vi "tb_push and pop random sequence.vi"(9 "fifo depth":u8(ring)=10 items=["4"=2, "8"=3, "16"=4, "32"=5, "64"=6, "128"=7, "256"=8, "512"=9, "1024"=10, "2048"=11, "4096"=12, "8192"=13, "16384"=14, "32768"=15, "65536"=16, "131072"=17, "262144"=18, "524288"=19, "1048576"=20, "2097152"=21, "4194304"=22, "8388608"=23, "16777216"=24, "33554432"=25, "67108864"=26, "134217728"=27, "268435456"=28, "536870912"=29, "1073741824"=30, "2147483648"=31, "4294967296"=32], 10 "arbiter configuration":T1={"write grant time (clocks)"=100, "read grant time (clocks)"=100}, 11 "Memory":T2={"fifo1 memory"="Bank0", "fifo2 memory"="Bank1"}) -> (3 "Pass?":bool=TRUE)   [LabVIEW 2011]
uses:
  Data Type (256).ctl
  <instrlib>/RF-RIO/Memory/FPGA/Interface/Timeslot Arbiter Configuration.ctl
  <instrlib>/RF-RIO/Memory/FPGA/Memory.lvlib
panel:
  out "Iteration":i32
  out "FIFO Input":T3[](array[typedef])
  out "FIFO Output":T3[](array[typedef])
  # "Debug Area"
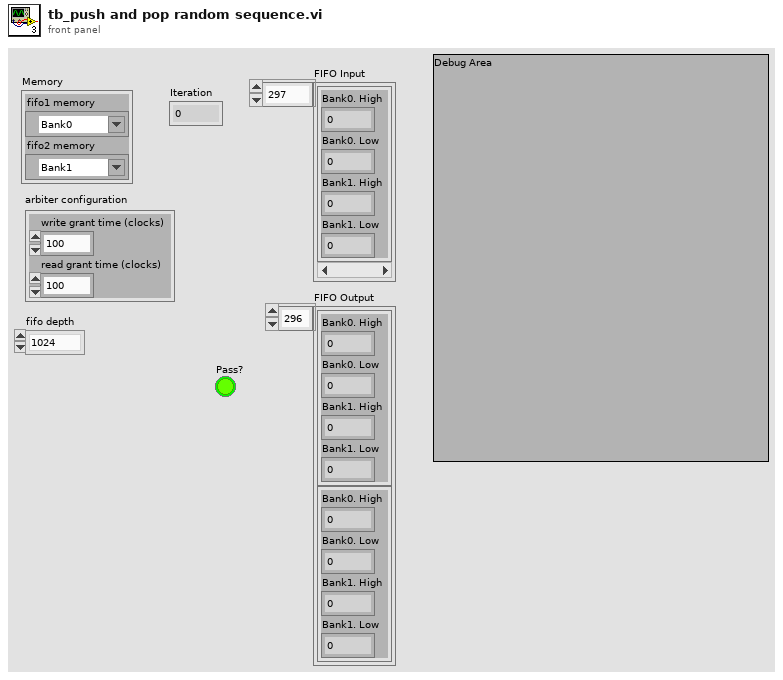
[diagram p1: front panel]
types:
  T1 = typedef "Memory.lvlib/Timeslot Arbiter Configuration.ctl" = cluster{"write grant time (clocks)":u16, "read grant time (clocks)":u16}
  T2 = cluster{"fifo1 memory":refnum<k21>, "fifo2 memory":refnum<k21>}
  T3 = typedef "Data Type (256).ctl" = cluster{"Bank0. High":u64, "Bank0. Low":u64, "Bank1. High":u64, "Bank1. Low":u64}
  T4 = cluster{"Bank0. High":bool, "Bank0. Low":bool, "Bank1. High":bool, "Bank1. Low":bool}[]
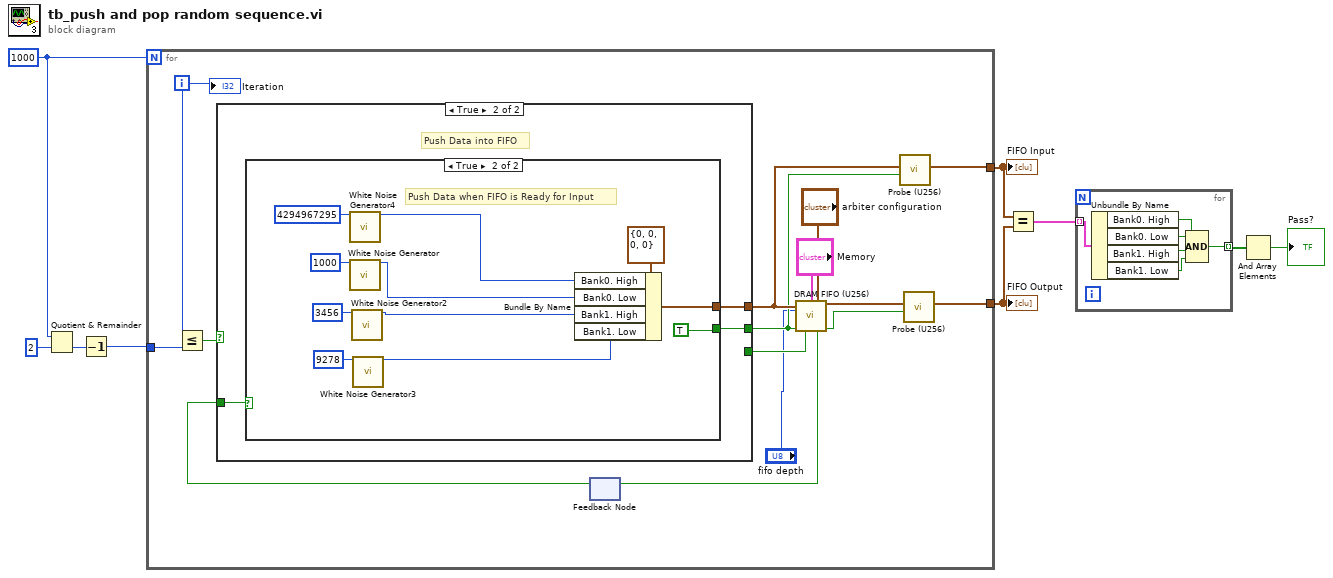
[diagram p0: block diagram]
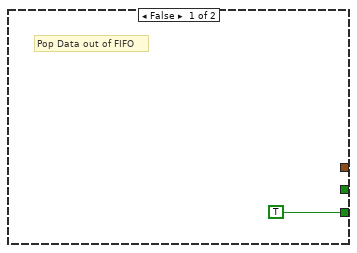
[diagram p2: hidden frame]
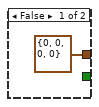
[diagram p3: hidden frame]
diagram:
  w9 = 1000
  n1 = Quotient & Remainder(x=w9, y=2) -> (floor(x/y)=w7:i32)  [unwired: 1 out]
  n2 = Decrement(x=w7) -> (x-1=w6:i32)
  n3 = for {
    N: w9 -> [_]
    tunnel: [w20] -> w4
    tunnel: [w17] -> w5
    tunnel: w6 -> [w14]
    i -> [w15]
    n4 = Less Or Equal?(x=w15, y=w14) -> (x <= y?=w16:bool)
    n5 = feedback #1() -> (w22:bool)  [unwired: 1 in]
    n6 = case shown="True" w16 {
      tunnel: [_ w28] -> w19
      tunnel: [_ w27] -> w18
      tunnel: w22 -> [_ w26]
      tunnel: [TRUE _] -> w21
      frame False {
        # "Pop Data out of FIFO"
      }
      frame True {
        # "Push Data into FIFO"
        n7 = case shown="True" w26 {
          tunnel: [T3 {"Bank0. High"=0, "Bank0. Low"=0, "Bank1. High"=0, "Bank1. Low"=0} ("Input Data") w39] -> w28
          tunnel: [_ TRUE] -> w27
          frame False {
          }
          frame True {
            # "Push Data when FIFO is Ready for Input"
            n8 = call "White Noise Generator4"("seed"=u32 4294967295) -> ("white noise out"=w30:i16)  [unwired: 14 in]
            n9 = call "White Noise Generator"("seed"=u32 1000) -> ("white noise out"=w31:i16)  [unwired: 14 in]
            n10 = call "White Noise Generator2"("seed"=u32 3456) -> ("white noise out"=w32:i16)  [unwired: 14 in]
            n11 = call "White Noise Generator3"("seed"=u32 9278) -> ("white noise out"=w33:i16)  [unwired: 14 in]
            n12 = Bundle By Name(cluster=T3 {"Bank0. High"=0, "Bank0. Low"=0, "Bank1. High"=0, "Bank1. Low"=0} ("Input Data"), "Bank0. High"=w30, "Bank0. Low"=w31, "Bank1. High"=w32, "Bank1. Low"=w33) -> (w39:T3)
          }
        }
      }
    }
    n13 = call "DRAM FIFO (U256).vi"("Input Data"=w19, "Memory"="Memory", "arbiter configuration"="arbiter configuration", "fifo depth"="fifo depth", "input valid"=w18, "ready for output"=w21) -> ("Output Data"=w11:T3, "Ready for Input"=w23:bool, "Output Valid"=w10:bool)  [unwired: 3 in, 4 out]
    n14 = feedback-in #1(w23) -> ()
    n15 = call "Probe (U256).vi"("Data Valid"=w18, "Input"=w19) -> ("Collected Data"=w17:T3[])  [unwired: 8 in, 1 out]
    n16 = call "Probe (U256).vi"("Data Valid"=w10, "Input"=w11) -> ("Collected Data"=w20:T3[])  [unwired: 8 in, 1 out]
    "Iteration" <- w15
  }
  "FIFO Output" <- w4
  "FIFO Input" <- w5
  n17 = Equal?(x=w5, y=w4) -> (x = y?=w3:T4)
  n18 = for {
    tunnel: w3 -> [w46] mode=indexing
    tunnel: [w41] -> w2 mode=indexing
    n19 = Unbundle By Name(w46) -> ("Bank0. High"=w45:bool, "Bank0. Low"=w44:bool, "Bank1. High"=w43:bool, "Bank1. Low"=w42:bool)
    n20 = Compound Arithmetic op=AND(w45, w44, w43, w42) -> (w41:bool)
  }
  n21 = And Array Elements(Boolean array=w2) -> (logical AND=→"Pass?":bool)
